vi "Education.vi"() -> ()   [LabVIEW 2021]
uses:
  <vilib>/Skyline/Tag/Shared/typedefs/DataType.ctl
  <vilib>/Skyline/Tag/Shared/NI Skyline Tag.lvlib
  <vilib>/Skyline/Tag/Wrapper/Wrapper HTTP_class/NI Skyline Tag HTTP.lvclass
  <vilib>/Skyline/Tag/Wrapper/Wrapper_class/NI Skyline Tag.lvclass
  <vilib>/Skyline/Configuration/Configuration HTTP_class/NI Skyline Configuration HTTP.lvclass
  <vilib>/Skyline/Configuration/Configuration HTTP_class/Open Configuration HTTP Auto.vi
  <vilib>/Skyline/Tag/Wrapper/Wrapper_class/Write Tag (I32).vi
panel:
  in  "stop":bool
  out "Amount donated (RON)":dbl
  out "Books bought":dbl
  in  "User Proposal prediction (only two classes possible: 0 or 1)":dbl
  out "AccuracyPrediction":dbl
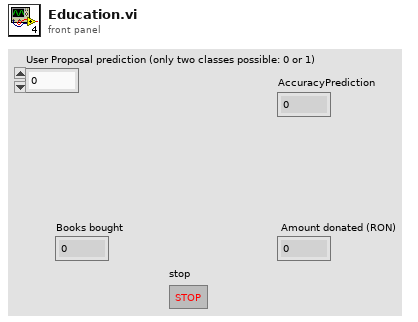
[diagram p1: front panel]
types:
  T1 = typedef "NI Skyline Tag.lvlib/DataType.ctl" = enum32{"Double", "I32", "String", "Boolean", "U64", "Timestamp"}
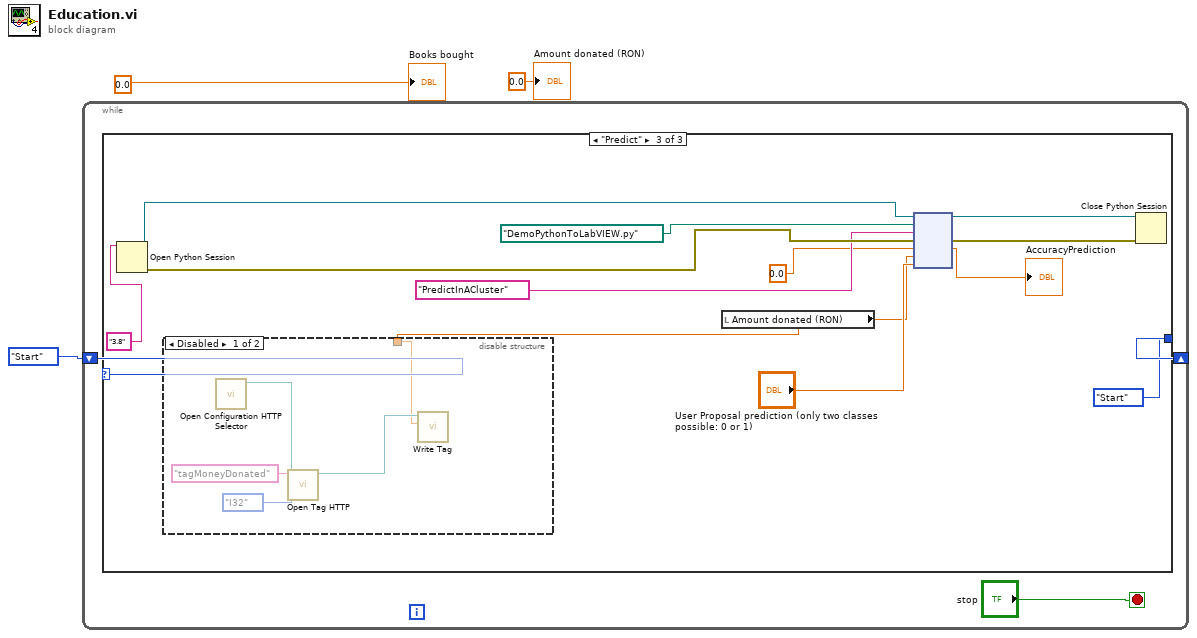
[diagram p0: block diagram]
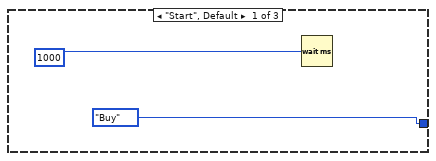
[diagram p2: hidden frame]
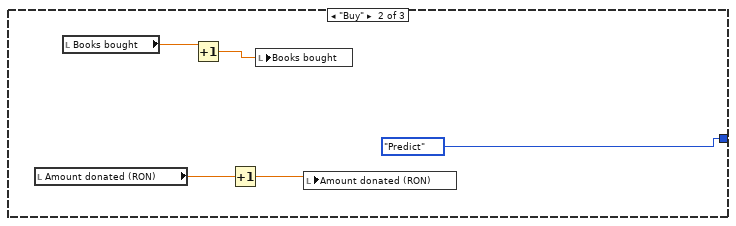
[diagram p3: hidden frame]
diagram:
  n1 = while {
    shift-right: [w5] -> _
    shift-left: enum16{"Start", "Buy", "Predict"}."Start" -> [w6]
    stop <- "stop" stop-if-true
    n2 = case shown="\"Predict\"" w6 {
      tunnel: [enum16{"Start", "Buy"}."Buy" enum16{"Start", "Buy", "Predict"}."Predict" enum16{"Start", "Buy", "Predict"}."Start"] -> w5
      frame "Start", Default {
        n3 = Wait (ms)(milliseconds to wait=u32 1000) -> ()  [unwired: 1 out]
      }
      frame "Buy" {
        n4 = local read "Amount donated (RON)"() -> (w10:dbl)
        n5 = local read "Books bought"() -> (w13:dbl)
        n6 = Increment(x=w13) -> (x+1=w12:dbl)
        n7 = Increment(x=w10) -> (x+1=w9:dbl)
        n8 = local write "Books bought"(w12) -> ()
        n9 = local write "Amount donated (RON)"(w9) -> ()
      }
      frame "Predict" {
        n10 = Open Python Session(python version="3.8" ("Python version")) -> (session out=w20:refnum<k35>, error out=w22:errorcluster)  [unwired: 2 in]
        n11 = local read "Amount donated (RON)"() -> (w14:dbl)
        n12 = disable-structure shown="Disabled" {
          disable-tunnel: w14 -> [w28 _]
          frame Disabled {
            n13 = call-poly <vilib>:"Open Configuration HTTP Selector.vi"() -> ("configuration"=w30:refnum<class "NI Skyline Configuration HTTP.lvclass">)  [unwired: 10 in, 1 out]
            n14 = call <vilib>:"Open Tag HTTP.vi"("configuration"=w30, "Data Type"=DataType."I32", "path"="tagMoneyDonated") -> ("tag"=w29:refnum<class "NI Skyline Tag.lvclass">)  [unwired: 7 in, 1 out]
            n15 = call-poly <vilib>:"Write Tag.vi"("value"=w28, "tag in"=w29) -> ()  [unwired: 8 in, 2 out]
          }
          frame Enabled {
          }
        }
        n16 = node(w20, path "DemoPythonToLabVIEW.py" ("module path"), "PredictInACluster" ("function name"), w22, 0.0, w14, "User Proposal prediction (only two classes possible: 0 or 1)") -> (w21:refnum<k35>, w23:errorcluster, →"AccuracyPrediction":dbl)  [unwired: 2 in, 2 out]
        n17 = Close Python Session(session in=w21, error in=w23) -> ()  [unwired: 1 out]
      }
    }
  }
  "Books bought" <- 0.0 ("Kg of food bought")
  "Amount donated (RON)" <- 0.0 ("Kg of food donated")
